vi "Initialize Session.vi"(8 "error in (no error)":errorcluster, 11 "Python Toolkit in":refnum<class "Python Toolkit.lvclass">) -> (0 "error out":errorcluster, 3 "Python Toolkit out":refnum<class "Python Toolkit.lvclass">)   [LabVIEW 2018, in "Python Toolkit.lvclass"]
uses:
  Python Toolkit.lvclass
  Python Toolkit.lvclass/Python Toolkit.ctl
  <vilib>/Enthought/Python Integration Toolkit/Python Integration Toolkit.lvlib
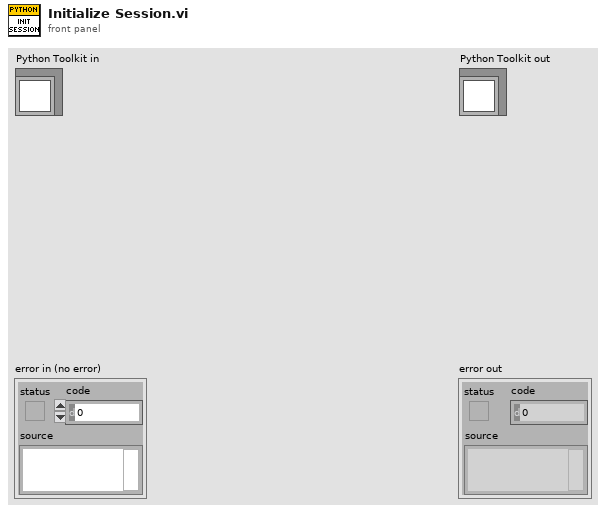
[diagram p1: front panel]
types:
  T1 = typedef "Python Integration Toolkit.lvlib/Session ID.ctl" = u64
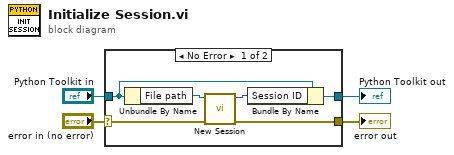
[diagram p0: block diagram]
diagram:
  n1 = case shown="No Error" "error in (no error)" {
    selector: "error in (no error)" -> [w10 w12]
    tunnel: [w9 w12] -> w3
    tunnel: [w6 w11] -> w1
    tunnel: "Python Toolkit in" -> [w7 w11]
    frame No Error {
      n2 = Unbundle By Name(w7) -> ("File path"=w8:path)
      n3 = call <vilib>:"New Session.vi"("error in (no error)"=w10, "Path to Python Module (.py File)"=w8) -> ("error out"=w9:errorcluster, "Session ID out"=w5:T1)  [unwired: 8 in]
      n4 = Bundle By Name(cluster=w7, "Session ID"=w5) -> (w6:refnum<class "Python Toolkit.lvclass">)
    }
    frame Error {
    }
  }
  "error out" <- w3
  "Python Toolkit out" <- w1
